vi "Init.vi"(8 "error in (no error)":errorcluster, 11 "Data Sharing Plugin Runtime.UDP in":refnum<class "Plugin Runtime.UDP.lvclass">) -> (0 "error out":errorcluster, 3 "Data Sharing Plugin Runtime.UDP out":refnum<class "Plugin Runtime.UDP.lvclass">)   [LabVIEW 2016, in "Plugin Runtime.UDP.lvclass"]
uses:
  Plugin Runtime.UDP.lvclass
  Plugin Runtime/Plugin Runtime.lvclass
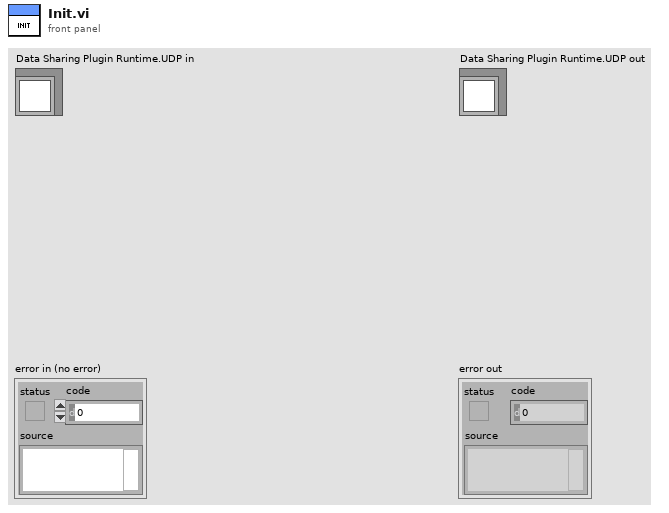
[diagram p1: front panel]
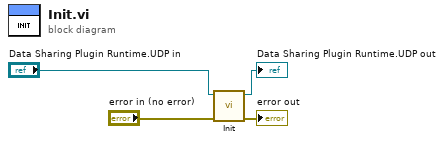
[diagram p0: block diagram]
diagram:
  n1 = call-parent "Init.vi"("error in (no error)"="error in (no error)", "Data Sharing Plugin Runtime in"="Data Sharing Plugin Runtime.UDP in") -> ("error out"=→"error out":errorcluster, "Data Sharing Plugin Runtime out"=→"Data Sharing Plugin Runtime.UDP out":refnum<class "Plugin Runtime.UDP.lvclass">)  [unwired: 8 in]
